vi "Init.vi"(8 "error in (no error)":errorcluster) -> (0 "error out":errorcluster, 3 "Game out":refnum<class "Game.lvclass">)   [LabVIEW 2020, in "SquareBattle.lvlib" / "Game.lvclass"]
uses:
  Game.lvclass
  Game.lvclass/Game.ctl
  Map/Map.lvclass
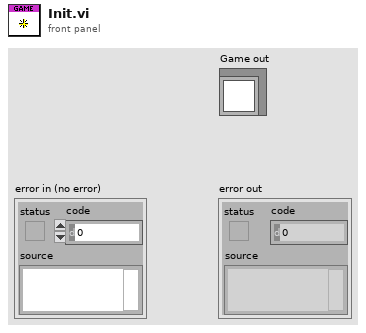
[diagram p1: front panel]
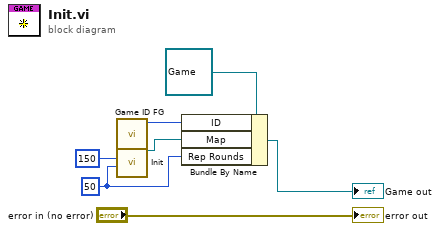
[diagram p0: block diagram]
diagram:
  w1 = u32 50 ("Replication Rounds")
  n1 = call "Game ID FG.vi"() -> ("Game ID"=w4:u16)  [unwired: 11 in]
  n2 = call "Init.vi"("Replication Rounds"=w1, "Size"=150) -> ("Map out"=w2:refnum<class "Map.lvclass">)  [unwired: 8 in, 1 out]
  n3 = Bundle By Name(cluster=refnum<class "Game.lvclass"> refnum ("Game in"), "ID"=w4, "Map"=w2, "Rep Rounds"=w1) -> (→"Game out":refnum<class "Game.lvclass">)
  "error out" <- "error in (no error)"
